vi "Launch New Display.vi"(8 "error in (no error)":errorcluster, 11 "Assert Startup UI in":refnum<class "Assert Startup UI.lvclass">) -> (0 "error out":errorcluster, 3 "Assert Startup UI out":refnum<class "Assert Startup UI.lvclass">)   [LabVIEW 2016, in "Assert API Components.lvlib" / "Assert Startup UI.lvlib" / "Assert Startup UI.lvclass"]
uses:
  Assert Startup UI.lvclass
  C:/Program Files (x86)/National Instruments/LabVIEW 2016/vi.lib/ActorFramework/Actor/Actor.lvclass
  Assert Display/Assert Display/Assert Display.lvclass/Assert Display.ctl
  Assert Startup UI.lvclass/Assert Startup UI.ctl
  Assert Display/Assert Display/Assert Display.lvclass
  <vilib>/ActorFramework/Actor/Actor.lvclass
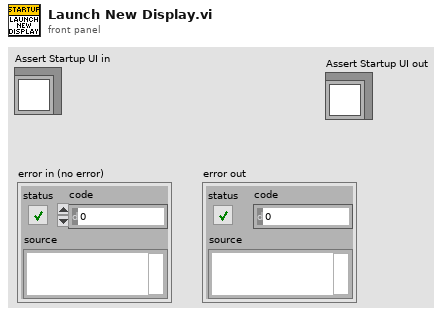
[diagram p1: front panel]
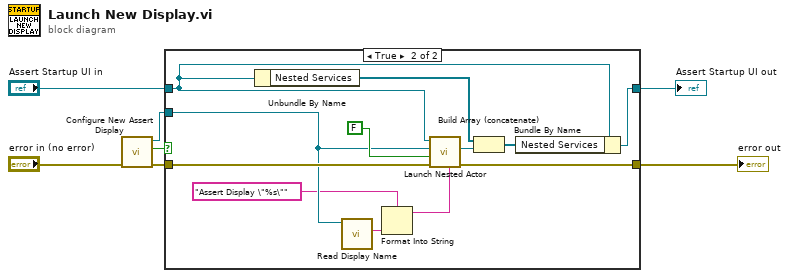
[diagram p0: block diagram]
diagram:
  n1 = call "Configure New Assert Display.vi"("error in (no error)"="error in (no error)") -> ("error out"=w5:errorcluster, "Build?"=w1:bool, "Assert Display out"=w4:refnum<class "Assert Display.lvclass">)  [unwired: 8 in]
  n2 = case shown="True" w1 {
    tunnel: [w8 w21] -> w7
    tunnel: w5 -> [w8 w20]
    tunnel: w4 -> [_ w13]
    tunnel: "Assert Startup UI in" -> [w9 w18]
    tunnel: [w9 w17] -> w2
    frame False {
    }
    frame True {
      n3 = Unbundle By Name(w18) -> ("Nested Services"=w19:refnum<class "Message Enqueuer.lvclass">[])
      n4 = call "Read Display Name.vi"("Assert Display in"=w13) -> ("Display Name"=w12:string)  [unwired: 10 in]
      n5 = Format Into String(format string="Assert Display \"%s\"", w12) -> (resulting string=w10:string)  [unwired: 2 in, 1 out]
      n6 = call <vilib>:"Launch Nested Actor.vi"("Debug Alias"=w10, "error in (no error)"=w20, "Auto-stop? (T)"=FALSE, "Nested Actor"=w13, "Caller Actor in"=w18) -> ("error out"=w21:errorcluster, "Nested Actor's Enqueuer"=w16:refnum<class "Message Enqueuer.lvclass">)  [unwired: 4 in, 1 out]
      n7 = Build Array (concatenate)(w19, w16) -> (w15:refnum<class "Message Enqueuer.lvclass">[])
      n8 = Bundle By Name(cluster=w18, "Nested Services"=w15) -> (w17:refnum<class "Assert Startup UI.lvclass">)
    }
  }
  "error out" <- w7
  "Assert Startup UI out" <- w2
